vi "CreateTriggerScanNode.vi"(7 "DOM Document":refnum<k20>, 8 "Error In":errorcluster, 11 "Trigger Scan Configuration":T1) -> (0 "Error Out":errorcluster, 3 "Trigger Scan Node":refnum<k20>)   [LabVIEW 2012]
uses:
  TriggerScanConfiguration.ctl
  driver/Public/Controls/ScanSource.ctl
  libs/LV-Utilities/LV-Utilities.lvlib
  driver/Keithley-7001.lvlib
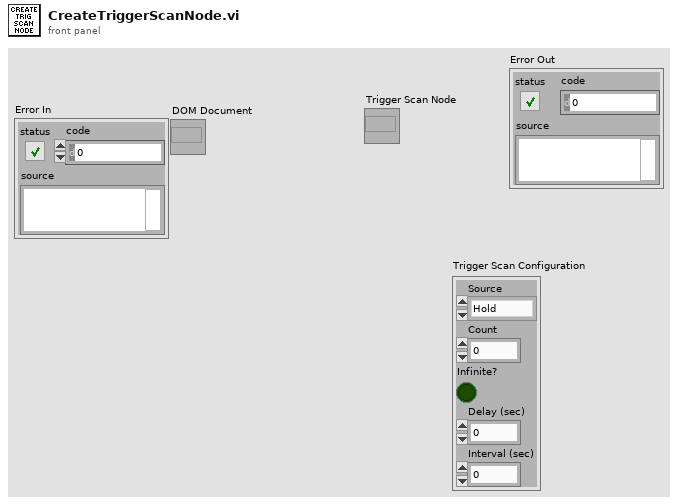
[diagram p1: front panel]
types:
  T1 = typedef "TriggerScanConfiguration.ctl" = cluster{"Source":T2, "Count":u32, "Infinite?":bool, "Delay (sec)":dbl, "Interval (sec)":dbl}
  T2 = typedef "Keithley-7001.lvlib/ScanSource.ctl" = enum16{"Hold", "Immediate", "Timer", "Manual", "Bus", "TLink", "External"}
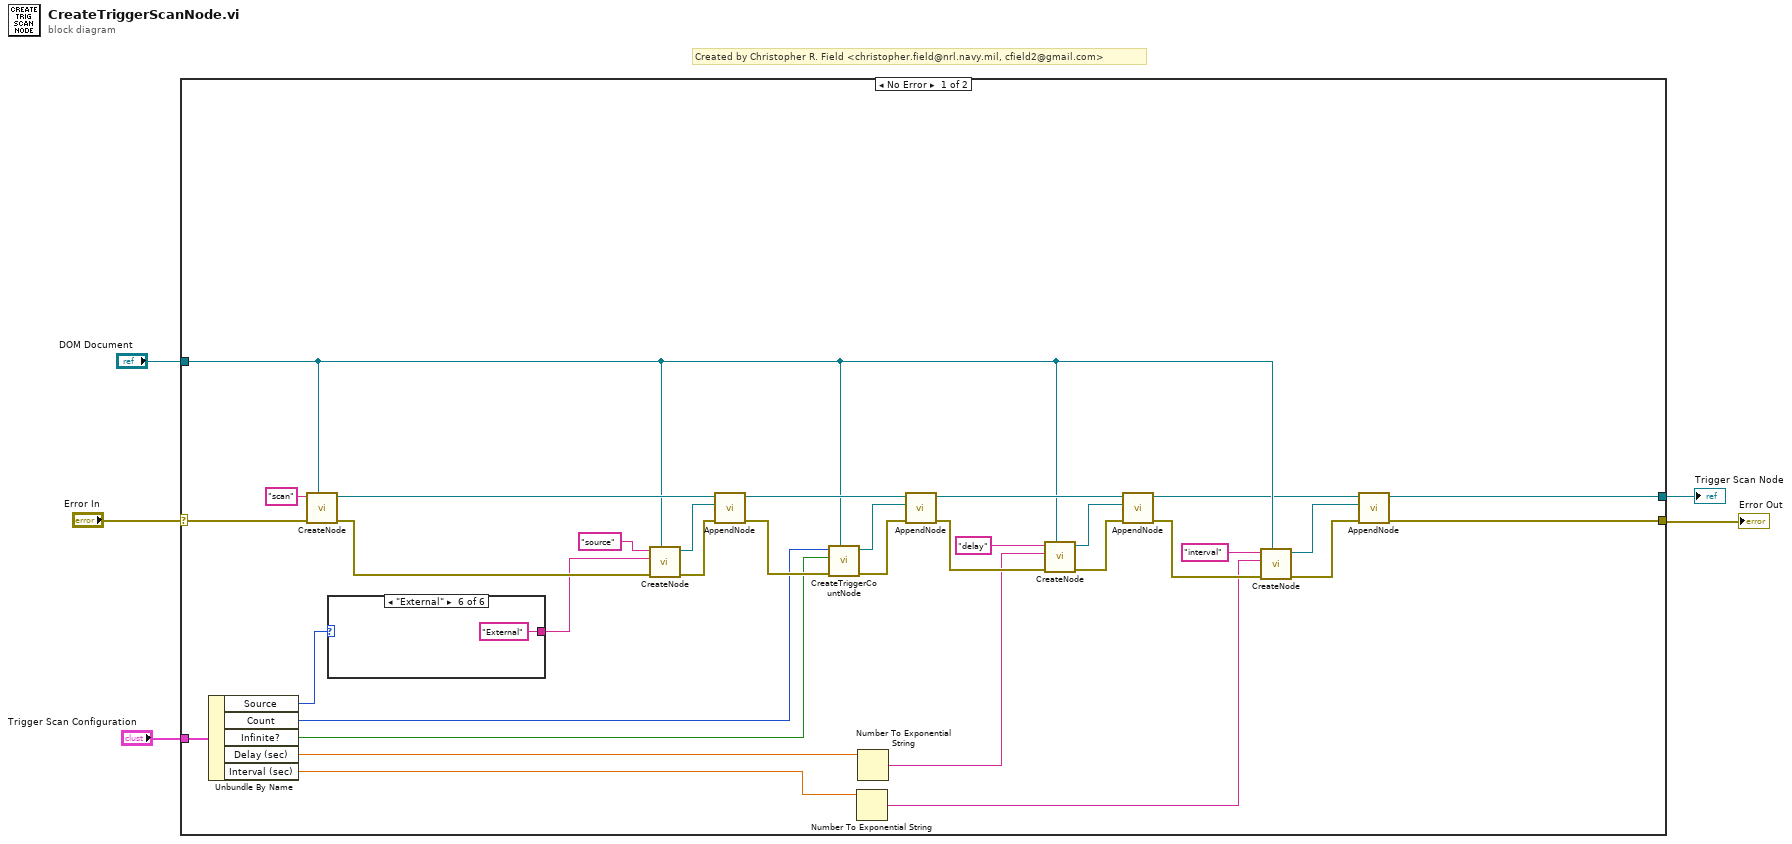
[diagram p0: block diagram]
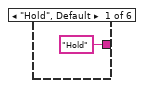
[diagram p2: hidden frame]
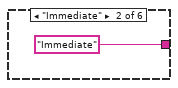
[diagram p3: hidden frame]
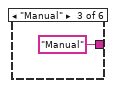
[diagram p4: hidden frame]
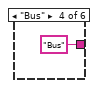
[diagram p5: hidden frame]
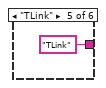
[diagram p6: hidden frame]
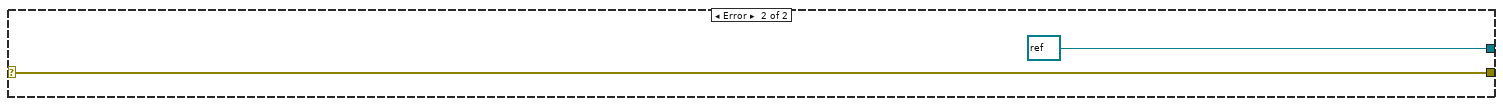
[diagram p7: hidden frame]
diagram:
  # "Created by Christopher R. Field <christopher.field@nrl.navy.mil, cfield2@gmail.com>"
  n1 = case shown="No Error" "Error In" {
    selector: "Error In" -> [w38 w46]
    tunnel: "DOM Document" -> [w11 _]
    tunnel: [w6 w46] -> w3
    tunnel: [w7 refnum<k20> refnum ("Wirings Node 2")] -> w2
    tunnel: "Trigger Scan Configuration" -> [w31 _]
    frame No Error {
      n2 = Unbundle By Name(w31) -> ("Source"=w30:T2, "Count"=w26:u32, "Infinite?"=w25:bool, "Delay (sec)"=w21:dbl, "Interval (sec)"=w15:dbl)
      n3 = call "CreateNode.vi"("DOM Document"=w11, "Error In"=w38, "Tag Name"="scan") -> ("Error out"=w35:errorcluster, "Node"=w34:refnum<k20>)  [unwired: 7 in]
      n4 = case shown="\"External\"" w30 {
        tunnel: ["Hold" "Immediate" "Manual" "Bus" "TLink" "External"] -> w29
        frame "Hold", Default {
        }
        frame "Immediate" {
        }
        frame "Manual" {
        }
        frame "Bus" {
        }
        frame "TLink" {
        }
        frame "External" {
        }
      }
      n5 = call "CreateNode.vi"("DOM Document"=w11, "Error In"=w35, "Text"=w29, "Tag Name"="source") -> ("Error out"=w33:errorcluster, "Node"=w32:refnum<k20>)  [unwired: 6 in]
      n6 = call "AppendNode.vi"("Error In"=w33, "Child Node"=w32, "Parent Node In"=w34) -> ("Error Out"=w27:errorcluster, "Parent Node Out"=w28:refnum<k20>)  [unwired: 7 in]
      n7 = call "CreateTriggerCountNode.vi"("DOM Document"=w11, "Error In"=w27, "Infinite?"=w25, "Count"=w26) -> ("Error Out"=w23:errorcluster, "Trigger Count Node"=w24:refnum<k20>)  [unwired: 6 in]
      n8 = Number To Exponential String(number=w15) -> (E-format string=w13:string)  [unwired: 3 in]
      n9 = Number To Exponential String(number=w21) -> (E-format string=w20:string)  [unwired: 3 in]
      n10 = call "AppendNode.vi"("Error In"=w23, "Child Node"=w24, "Parent Node In"=w28) -> ("Error Out"=w22:errorcluster, "Parent Node Out"=w18:refnum<k20>)  [unwired: 7 in]
      n11 = call "CreateNode.vi"("DOM Document"=w11, "Error In"=w22, "Text"=w20, "Tag Name"="delay") -> ("Error out"=w16:errorcluster, "Node"=w17:refnum<k20>)  [unwired: 6 in]
      n12 = call "AppendNode.vi"("Error In"=w16, "Child Node"=w17, "Parent Node In"=w18) -> ("Error Out"=w14:errorcluster, "Parent Node Out"=w10:refnum<k20>)  [unwired: 7 in]
      n13 = call "CreateNode.vi"("DOM Document"=w11, "Error In"=w14, "Text"=w13, "Tag Name"="interval") -> ("Error out"=w9:errorcluster, "Node"=w8:refnum<k20>)  [unwired: 6 in]
      n14 = call "AppendNode.vi"("Error In"=w9, "Child Node"=w8, "Parent Node In"=w10) -> ("Error Out"=w6:errorcluster, "Parent Node Out"=w7:refnum<k20>)  [unwired: 7 in]
    }
    frame Error {
    }
  }
  "Trigger Scan Node" <- w2
  "Error Out" <- w3
